vi "Test Leap Code.vi"() -> ()   [LabVIEW 2014]
uses:
  <vilib>/MakerHub/Leap/LMH-Leap.lvlib
panel:
  out "find list":string[](array[string])
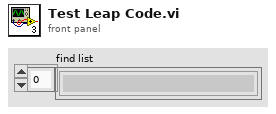
[diagram p1: front panel]
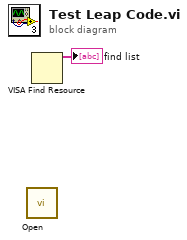
[diagram p0: block diagram]
diagram:
  n1 = call <vilib>:"Open.vi"() -> ()  [unwired: 10 in, 2 out]
  n2 = VISA Find Resource() -> (3:→"find list":string[])  [unwired: 3 in, 2 out]
